vi "Filter Versions_strings.vi"(8 "error in (no error)":errorcluster, 10 "Version Range":string, 11 "Semver Strings":string[](array[string])) -> (0 "error out":errorcluster, 2 "Pointers":i32[](array[numeric]), 3 "Filtered Semvers":refnum<class "Semver.lvclass">[](array[class]))   [LabVIEW 2017, in "Semver.lvlib" / "Semver.lvclass"]
uses:
  Semver.lvclass
  Semver.lvclass/Semver.ctl
  Parse Number.vi
  <vilib>/Utility/error.llb/Error Cluster From Error Code.vi
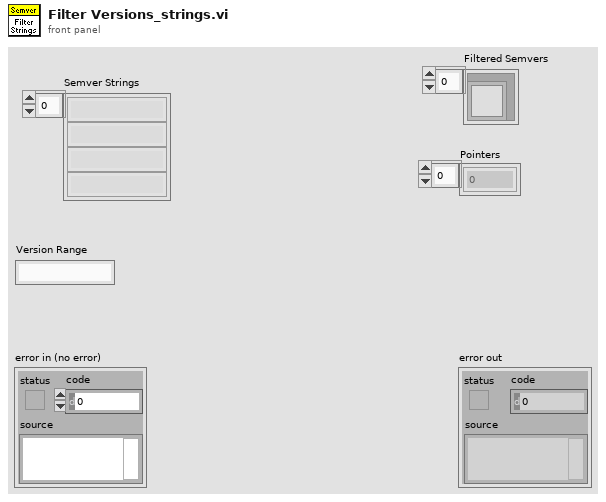
[diagram p1: front panel]
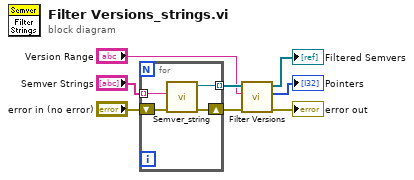
[diagram p0: block diagram]
diagram:
  n1 = for {
    shift-right: [w11] -> w5
    shift-left: "error in (no error)" -> [w12]
    tunnel: "Semver Strings" -> [w10] mode=indexing
    tunnel: [w9] -> w6 mode=indexing
    n2 = call "Semver_string.vi"("error in (no error)"=w12, "Version"=w10) -> ("error out"=w11:errorcluster, "Semver out"=w9:refnum<class "Semver.lvclass">)  [unwired: 8 in]
  }
  n3 = call "Filter Versions.vi"("error in (no error)"=w5, "Version Range"="Version Range", "Semvers in"=w6) -> ("error out"=→"error out":errorcluster, "Pointers"=→"Pointers":i32[], "Filtered Semvers"=→"Filtered Semvers":refnum<class "Semver.lvclass">[])  [unwired: 6 in]
